vi "Azimut and FOV Calibration.vi"(0 "Main Interface":T1, 1 "Manipulator Interface":T6, 2 "Calibration":T3, 3 "Parameters":enum16{"Azimut", "FOV", "Azimut and FOV"}(ring), 4 "Focus and Tracking":T2, 5 "Error In":errorcluster, 6 "Distance [um]":dbl, 7 "System of Reference Interface":T5, 8 "Initial [pix]":cluster{"X":sgl, "Y":sgl}, 9 "Diagonal factor":dbl=0.5 min=0.0 max=1.0, 10 "Final [pix]":cluster{"X":sgl, "Y":sgl}, 11 "Initial Reference [um]":T4, 13 "Final Reference [um]":T4) -> (19 "Error Out":errorcluster)   [LabVIEW 2012, in "Targeting Unit.lvlib"]
uses:
  Targeting Unit.lvlib
  <vilib>/Analysis/Matrix/Datatypes/RealMatrix.ctl
  <vilib>/Analysis/Matrix/NI_Matrix.lvlib
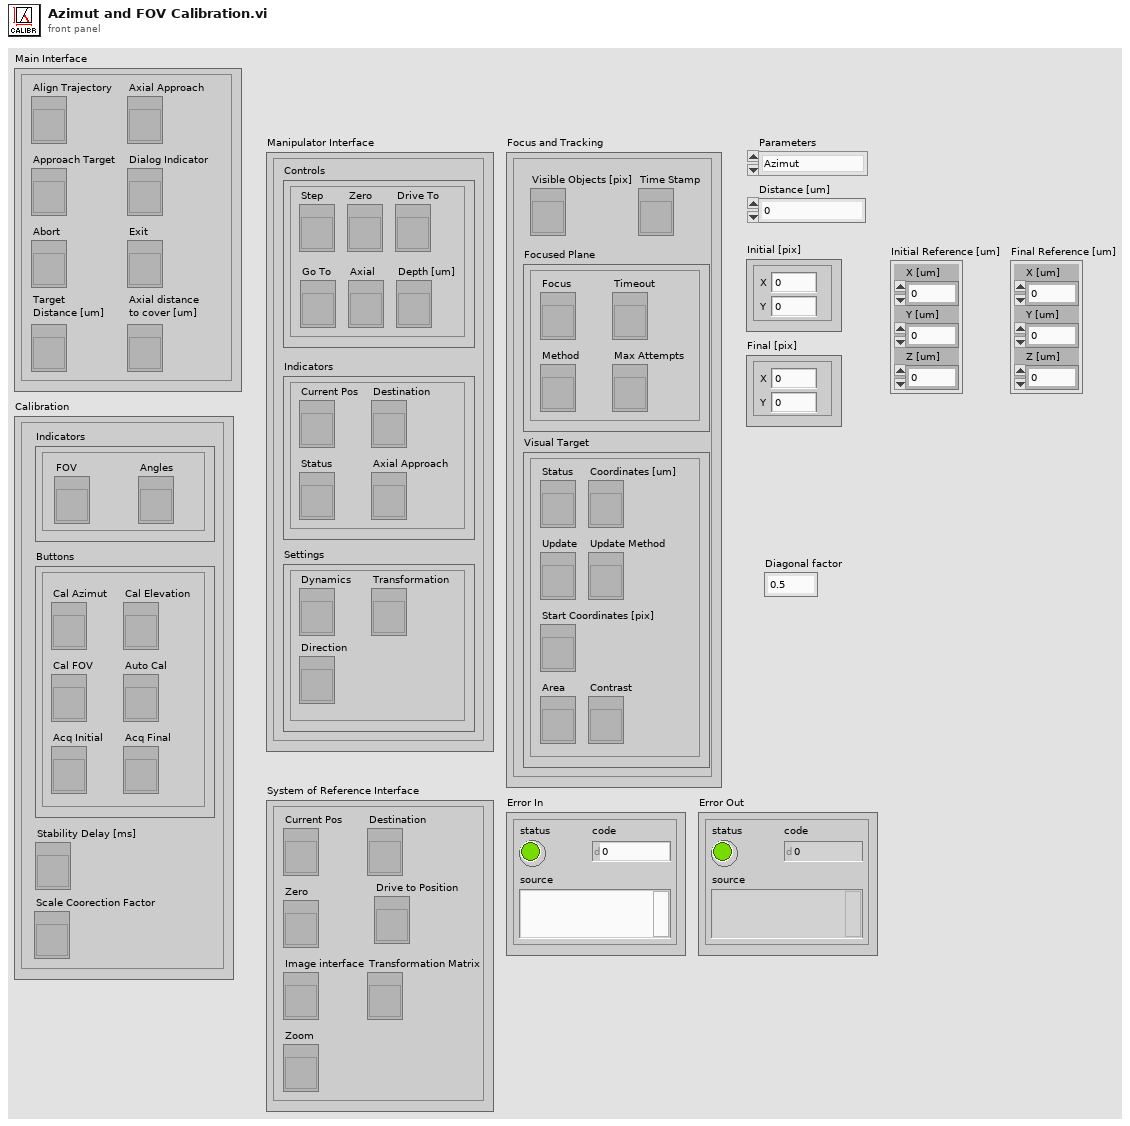
[diagram p1: front panel]
types:
  T1 = cluster{"Exit":refnum<vi>, "Abort":refnum<vi>, "Align Trajectory":refnum<vi>, "Axial Approach":refnum<vi>, "Dialog Indicator":refnum<vi>, "Approach Target":refnum<vi>, "Target\nDistance [um]":refnum<vi>, "Axial distance\nto cover [um]":refnum<vi>}
  T2 = cluster{"Focused Plane":cluster{"Focus":refnum<vi>, "Timeout":refnum<vi>, "Max Attempts":refnum<vi>, "Method":refnum<vi>}, "Time Stamp":refnum<vi>, "Visual Target":cluster{"Coordinates [um]":refnum<vi>, "Status":refnum<vi>, "Update":refnum<vi>, "Update Method":refnum<vi>, "Start Coordinates [pix]":refnum<vi>, "Area":refnum<vi>, "Contrast":refnum<vi>}, "Visible Objects [pix]":refnum<vi>}
  T3 = cluster{"Indicators":cluster{"FOV":refnum<vi>, "Angles":refnum<vi>}, "Buttons":cluster{"Cal FOV":refnum<vi>, "Cal Azimut":refnum<vi>, "Cal Elevation":refnum<vi>, "Auto Cal":refnum<vi>, "Acq Initial":refnum<vi>, "Acq Final":refnum<vi>}, "Stability Delay [ms]":refnum<vi>, "Scale Coorection Factor":refnum<vi>}
  T4 = cluster{"X [um]":dbl, "Y [um]":dbl, "Z [um]":dbl}
  T5 = cluster{"Current Pos":refnum<vi>, "Image interface":refnum<vi>, "Transformation Matrix":refnum<vi>, "Zero":refnum<vi>, "Destination":refnum<vi>, "Drive to Position":refnum<vi>, "Zoom":refnum<vi>}
  T6 = cluster{"Indicators":cluster{"Current Pos":refnum<vi>, "Destination":refnum<vi>, "Status":refnum<vi>, "Axial Approach":refnum<vi>}, "Settings":cluster{"Dynamics":refnum<vi>, "Transformation":refnum<vi>, "Direction":refnum<vi>}, "Controls":cluster{"Zero":refnum<vi>, "Step":refnum<vi>, "Drive To":refnum<vi>, "Go To":refnum<vi>, "Axial":refnum<vi>, "Depth [um]":refnum<vi>}}
  T7 = typedef "NI_Matrix.lvlib/RealMatrix.ctl" = dbl[][]
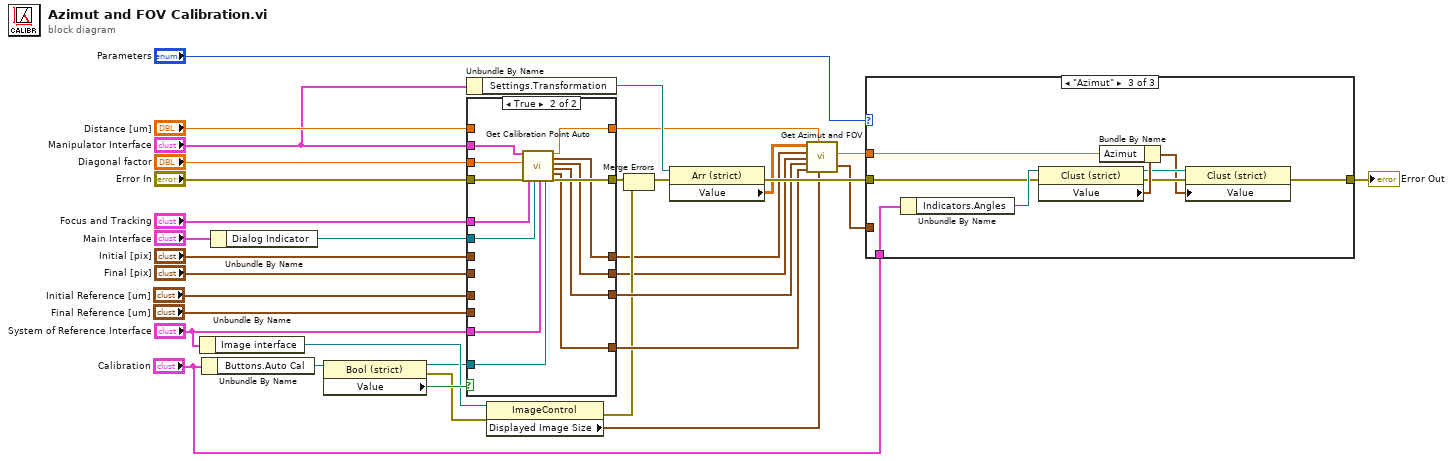
[diagram p0: block diagram]
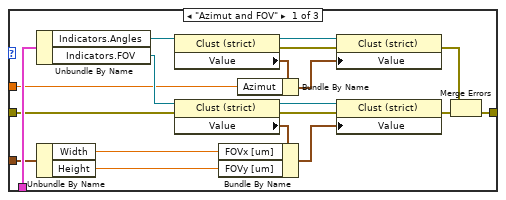
[diagram p2: hidden frame]
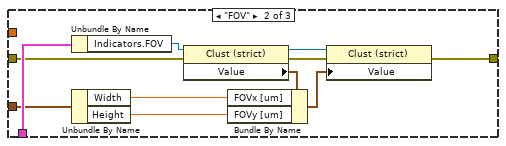
[diagram p3: hidden frame]
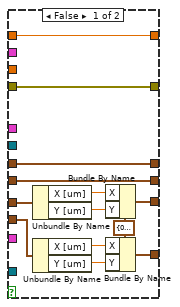
[diagram p4: hidden frame]
diagram:
  n1 = Unbundle By Name("System of Reference Interface") -> ("Image interface"=w12:refnum<vi>)
  n2 = Unbundle By Name("Calibration") -> ("Buttons.Auto Cal"=w23:refnum<vi>)
  n3 = Unbundle By Name("Main Interface") -> ("Dialog Indicator"=w33:refnum<vi>)
  n4 = property class="Bool (strict)"(reference=w23) -> (reference out=w8:refnum<vi>, error out=w10:errorcluster, "Value"=w22:bool)  [unwired: 1 in]
  n5 = Unbundle By Name("Manipulator Interface") -> ("Settings.Transformation"=w31:refnum<vi>)
  n6 = case shown="True" w22 {
    tunnel: "Manipulator Interface" -> [_ w60]
    tunnel: "Error In" -> [w46 w59]
    tunnel: w33 -> [_ w51]
    tunnel: "Diagonal factor" -> [_ w58]
    tunnel: "Focus and Tracking" -> [_ w50]
    tunnel: [w47 w57] -> w19
    tunnel: [w46 w56] -> w21
    tunnel: "Initial [pix]" -> [w45 _]
    tunnel: "Final [pix]" -> [w44 _]
    tunnel: "Distance [um]" -> [w47 _]
    tunnel: w8 -> [_ w52]
    tunnel: [w39 w54] -> w16
    tunnel: [w38 w53] -> w15
    tunnel: "System of Reference Interface" -> [_ w55]
    tunnel: [w45 w49] -> w7
    tunnel: [w44 w48] -> w6
    tunnel: "Initial Reference [um]" -> [w36 _]
    tunnel: "Final Reference [um]" -> [w35 _]
    frame False {
      w37 = cluster{"X":dbl, "Y":dbl} {"X"=0.0, "Y"=0.0} ("Initial Reference Point [um]")
      n7 = Unbundle By Name(w36) -> ("X [um]"=w42:dbl, "Y [um]"=w43:dbl)
      n8 = Unbundle By Name(w35) -> ("X [um]"=w41:dbl, "Y [um]"=w40:dbl)
      n9 = Bundle By Name(cluster=w37, "X"=w42, "Y"=w43) -> (w39:cluster{"X":dbl, "Y":dbl})
      n10 = Bundle By Name(cluster=w37, "X"=w41, "Y"=w40) -> (w38:cluster{"X":dbl, "Y":dbl})
    }
    frame True {
      n11 = call "Get Calibration Point Auto.vi"("Manipulator Interface"=w60, "Diagonal factor"=w58, "Focus and Tracking"=w50, "error in"=w59, "System of Reference Interface"=w55, "Dialog Indicator"=w51, "Calibrate button"=w52) -> ("Distance [um]"=w57:dbl, "Initial [pix]"=w49:cluster{"X":sgl, "Y":sgl}, "Final [pix]"=w48:cluster{"X":sgl, "Y":sgl}, "Initial Reference Point [um]"=w54:cluster{"X":dbl, "Y":dbl}, "Final Reference Point [um]"=w53:cluster{"X":dbl, "Y":dbl}, "error out"=w56:errorcluster)  [unwired: 7 in]
    }
  }
  n12 = property class="ImageControl"(reference=w12, error in=w10) -> (error out=w9:errorcluster, "Displayed Image Size"=w13:cluster{"Width":u32, "Height":u32})  [unwired: 1 out]
  n13 = Merge Errors(w21, w9) -> (w20:errorcluster)
  n14 = property class="Arr (strict)"(reference=w31, error in=w20) -> (error out=w29:errorcluster, "Value"=w14:T7)  [unwired: 1 out]
  n15 = call "Get Azimut and FOV.vi"("Transformation Matrix"=w14, "Image Size [pix]"=w13, "Axial Distance [um]"=w19, "Final Reference Point [um]"=w15, "Initial Reference Point [um]"=w16, "Final Visual Point[pix]"=w6, "Initial Visual Point [pix]"=w7) -> ("Angle [rad]"=w17:dbl, "FOV [um]"=w18:cluster{"Width":dbl, "Height":dbl})  [unwired: 2 in, 1 out]
  n16 = case shown="\"Azimut\"" "Parameters" {
    tunnel: "Calibration" -> [w67 w90 w97]
    tunnel: w18 -> [w66 w81 _]
    tunnel: w17 -> [w65 _ w95]
    tunnel: w29 -> [w64 w82 w93]
    tunnel: [w61 w80 w91] -> w28
    frame "Azimut and FOV" {
      n17 = Unbundle By Name(w67) -> ("Indicators.Angles"=w79:refnum<vi>, "Indicators.FOV"=w74:refnum<vi>)
      n18 = Unbundle By Name(w66) -> ("Width"=w72:dbl, "Height"=w71:dbl)
      n19 = property class="Clust (strict)"(reference=w79) -> (reference out=w75:refnum<vi>, error out=w78:errorcluster, "Value"=w76:cluster{"Azimut":dbl, "Elevation":dbl})  [unwired: 1 in]
      n20 = property class="Clust (strict)"(reference=w74, error in=w64) -> (reference out=w69:refnum<vi>, error out=w70:errorcluster, "Value"=w73:cluster{"FOVx [um]":dbl, "FOVy [um]":dbl})
      n21 = Bundle By Name(cluster=w73, "FOVx [um]"=w72, "FOVy [um]"=w71) -> (w68:cluster{"FOVx [um]":dbl, "FOVy [um]":dbl})
      n22 = Bundle By Name(cluster=w76, "Azimut"=w65) -> (w77:cluster{"Azimut":dbl, "Elevation":dbl})
      n23 = property class="Clust (strict)"(reference=w75, error in=w78, "Value"=w77) -> (error out=w62:errorcluster)  [unwired: 1 out]
      n24 = property class="Clust (strict)"(reference=w69, error in=w70, "Value"=w68) -> (error out=w63:errorcluster)  [unwired: 1 out]
      n25 = Merge Errors(w62, w63) -> (w61:errorcluster)
    }
    frame "FOV" {
      n26 = Unbundle By Name(w90) -> ("Indicators.FOV"=w89:refnum<vi>)
      n27 = Unbundle By Name(w81) -> ("Width"=w87:dbl, "Height"=w86:dbl)
      n28 = property class="Clust (strict)"(reference=w89, error in=w82) -> (reference out=w84:refnum<vi>, error out=w85:errorcluster, "Value"=w88:cluster{"FOVx [um]":dbl, "FOVy [um]":dbl})
      n29 = Bundle By Name(cluster=w88, "FOVx [um]"=w87, "FOVy [um]"=w86) -> (w83:cluster{"FOVx [um]":dbl, "FOVy [um]":dbl})
      n30 = property class="Clust (strict)"(reference=w84, error in=w85, "Value"=w83) -> (error out=w80:errorcluster)  [unwired: 1 out]
    }
    frame "Azimut" {
      n31 = Unbundle By Name(w97) -> ("Indicators.Angles"=w98:refnum<vi>)
      n32 = property class="Clust (strict)"(reference=w98, error in=w93) -> (reference out=w96:refnum<vi>, error out=w94:errorcluster, "Value"=w99:cluster{"Azimut":dbl, "Elevation":dbl})
      n33 = Bundle By Name(cluster=w99, "Azimut"=w95) -> (w92:cluster{"Azimut":dbl, "Elevation":dbl})
      n34 = property class="Clust (strict)"(reference=w96, error in=w94, "Value"=w92) -> (error out=w91:errorcluster)  [unwired: 1 out]
    }
  }
  "Error Out" <- w28
